vi "Collapse Menu.vi"(8 "error in (no error)":errorcluster, 11 "MenuButton in":refnum<class "MenuButton.lvclass">) -> (0 "error out":errorcluster, 2 "Menu Bottom Position":u32, 3 "MenuButton out":refnum<class "MenuButton.lvclass">)   [LabVIEW 2017, in "MenuButtons.lvlib" / "MenuButton.lvclass"]
uses:
  MenuButton.lvclass
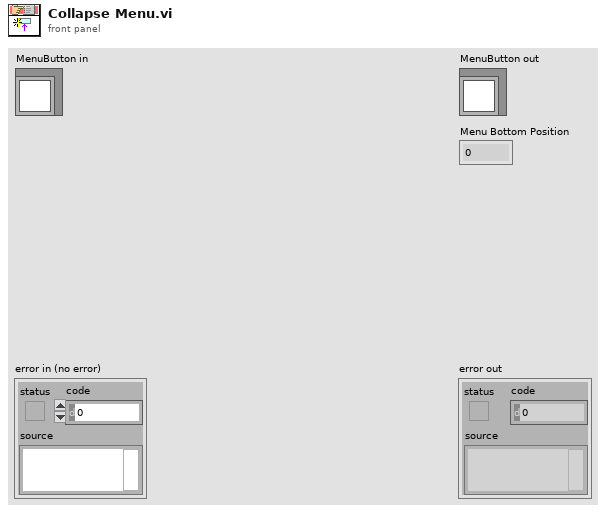
[diagram p1: front panel]
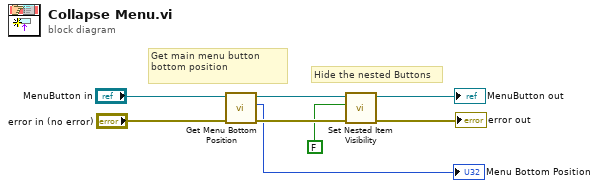
[diagram p0: block diagram]
diagram:
  # "Get main menu button bottom position"
  # "Hide the nested Buttons"
  n1 = call "Get Menu Bottom Position.vi"("error in (no error)"="error in (no error)", "MenuButton in"="MenuButton in") -> ("error out"=w4:errorcluster, "Menu Bottom Position"=→"Menu Bottom Position":u32, "MenuButton out"=w8:refnum<class "MenuButton.lvclass">)  [unwired: 7 in]
  n2 = call "Set Nested Item Visibility.vi"("error in (no error)"=w4, "Visible?"=FALSE, "MenuButton in"=w8) -> ("error out"=→"error out":errorcluster, "MenuButton out"=→"MenuButton out":refnum<class "MenuButton.lvclass">)  [unwired: 7 in]
